vi "draw Fz.vi"(11 "FZ":dbl[][][](array[numeric])) -> (3 "X_Y_Plot":cluster{"x":dbl[], "y":dbl[]}[](array[cluster]))   [LabVIEW 2019]
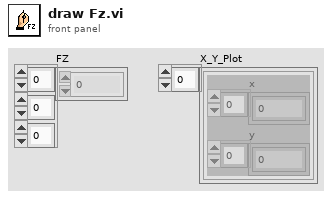
[diagram p1: front panel]
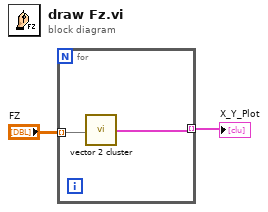
[diagram p0: block diagram]
diagram:
  n1 = for {
    tunnel: "FZ" -> [w4] mode=indexing
    tunnel: [w3] -> w2 mode=indexing
    n2 = call "vector 2 cluster.vi"("coordinates"=w4) -> (0:w3:cluster{"x":dbl[], "y":dbl[]})
  }
  "X_Y_Plot" <- w2
